vi "Untitled 1.vi"() -> ()   [LabVIEW 2017]
uses:
  <vilib>/visionFPGA/Controls/IMAQ FPGA Image Size.ctl
  <vilib>/Platform/TimedLoop/XDataNode/timing_clust.ctl
  <vilib>/Platform/TimedLoop/XDataNode/nitl_modes.ctl
  <vilib>/Platform/TimedLoop/XDataNode/wakeup.ctl
  <vilib>/rvi/Emulation/niFpgaSctlEmulationGetInTimedLoop.vi
  <vilib>/rvi/Emulation/niFpgaEmulationReportErrorSimple.vi
  <vilib>/rvi/Emulation/niFpgaGetClockAttributes.vi
  <vilib>/rvi/Emulation/niFpgaCriticalErrorInLSC.vi
  <vilib>/visionFPGA/Basics/FIFO to Pixel Bus/IMAQ FPGA FIFO to Pixel Bus U8x1.vi
  <vilib>/visionFPGA/Basics/Pixel Bus to FIFO/IMAQ FPGA Pixel Bus to FIFO U1x1.vi
  <vilib>/platform/TimedLoop/XDataNode/XDataNode.xnode
  <vilib>/Platform/TimedLoop/XDataNode/XDNodeRunTimeDep.lvlib
  <vilib>/visionFPGA/NI_VDM_FPGA_Basics.lvlib
panel:
  in  "Image Size":T1
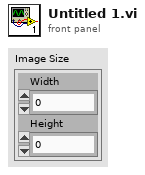
[diagram p1: front panel]
types:
  T1 = typedef "IMAQ FPGA Image Size.ctl" = cluster{"Width":u32, "Height":u32}
  T2 = typedef "XDNodeRunTimeDep.lvlib/timing_clust.ctl" = cluster{"Expected End [f-1]":u64, "Actual End [f-1]":u64, "Finished Late? [f-1]":bool, "Expected End [i-1]":u64, "Actual End [i-1]":u64, "Finished Late? [i-1]":bool, "Expected Start [i]":u64, "Actual Start [i]":u64, "Expected Start [f]":u64, "Actual Start [f]":u64, "Source Name":string, "Structure Name":string, "Period":i64, "Deadline":i64, "Offset":i64, "Start":i64, "Priority":i32, "Timeout":i32, "Mode":T3, "Wakeup Reason":T4, "Error":errorcluster, "Source Type":string, "Secondary Source Type":string, "Global End Time":u64, "Global Start Time":u64, "Frame Duration":u64, "Iteration Duration":u64, "Assigned CPU":i32, "I/O Scan Engine Mode":u32}
  T3 = typedef "XDNodeRunTimeDep.lvlib/nitl_modes.ctl" = enum32{"No Change", "Process missed periods, maintain original phase", "Discard missed periods, maintain original phase", "Process missed periods, ignore original phase", "Discard missed periods, ignore original phase"}
  T4 = typedef "XDNodeRunTimeDep.lvlib/wakeup.ctl" = enum32{"Normal", "Aborted", "Asynchronous wakeup", "Timing source error", "Timed loop error", "Timeout"}
  T5 = typedef "IMAQ FPGA Pixel Bus u8x1.ctl" = cluster{"Pixel Data":u8, "DV":bool, "EOL":bool, "EOI":bool, "Data Type":enum16{"U8 x 1"}}
  T6 = typedef "IMAQ FPGA Pixel Bus u1x1.ctl" = cluster{"Pixel Data":bool, "DV":bool, "EOL":bool, "EOI":bool, "Data Type":enum16{"U1 x 1"}}
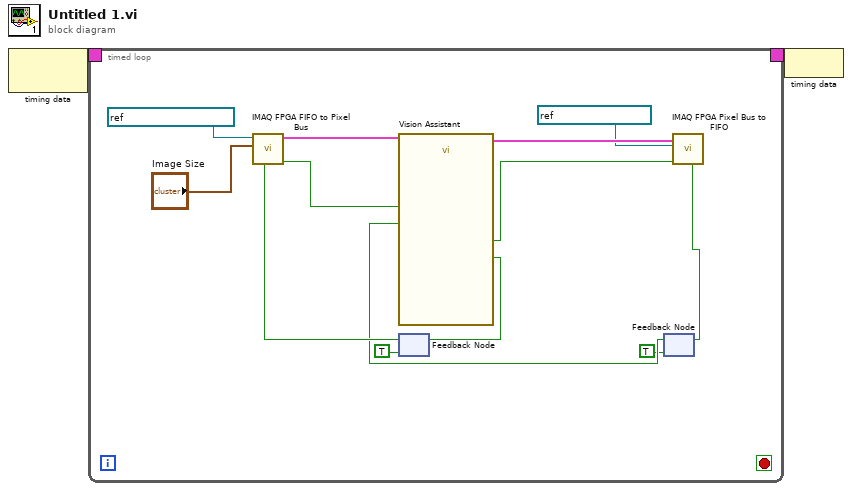
[diagram p0: block diagram]
diagram:
  n1 = node-c288() -> (w2:T2)  [unwired: 1 in]
  n2 = timed-loop {
    timing: w2 -> [_]
    timing-out: [_] -> w1
    stop <- _ stop-if-true
    n3 = feedback #1(TRUE ("Ready for Input")) -> (w10:bool)
    n4 = call-poly <vilib>:"IMAQ FPGA FIFO to Pixel Bus.vi"("Ready For Output"=w10, "Image Size"="Image Size", "Source Image FIFO"=refnum<k21> "Source Image FIFO") -> ("Output Valid"=w12:bool, "Pixel Bus Out"=w13:T5)  [unwired: 6 in, 1 out]
    n5 = feedback #2(TRUE ("Ready for Input")) -> (w4:bool)
    n6 = call "Vision Assistant"("Pixel Bus"=w13, "Input Valid"=w12, "Ready for Output"=w4) -> ("Ready for Input"=w11:bool, "Pixel Bus Out"=w8:T6, "Output Valid"=w7:bool)  [unwired: 21 in, 1 out]
    n7 = feedback-in #1(w11) -> ()
    n8 = call-poly <vilib>:"IMAQ FPGA Pixel Bus to FIFO.vi"("Input Valid"=w7, "Destination Image FIFO"=refnum<k21> "Dest Image FIFO", "Pixel Bus In"=w8) -> ("Ready for Input"=w5:bool)  [unwired: 8 in]
    n9 = feedback-in #2(w5) -> ()
  }
  n10 = node-c288(w1) -> ()
